vi "Add Item to Tree.vi"(8 "error in (no error)":errorcluster, 10 "Missing VI Type in":refnum<class "Missing VI Type.lvclass">, 11 "Tree Ref in":refnum<vi>) -> (0 "error out":errorcluster, 1 "Added Tag":string, 2 "Missing VI Type out":refnum<class "Missing VI Type.lvclass">, 3 "Tree Ref out":refnum<vi>)   [LabVIEW 2020, in "Peek Window.lvlib" / "Missing VI Type.lvclass"]
uses:
  Missing VI Type.lvclass
  D:/Code/VI-Peek/source/Peek Window/VI Types/Standard VI Type/Standard VI Type.lvclass
  Symbols Enum.ctl
  Standard VI Type/Standard VI Type.lvclass/Standard VI Type.ctl
  Standard VI Type/Read Full Qualified Name.vi
  Peek Window.lvlib
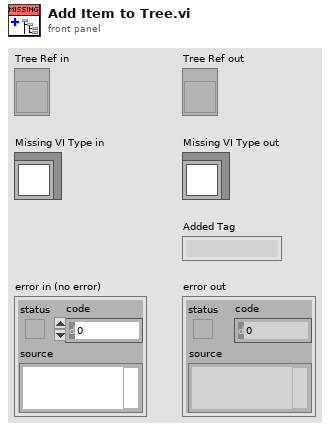
[diagram p1: front panel]
types:
  T1 = typedef "Peek Window.lvlib/Symbols Enum.ctl" = enum16{"<Blank>", "Below Here Glyph", "VI", "Dynamic Dispatch VI", "Malleable VI", "Polymorphic VI", "Missing VI", "Express VI"}
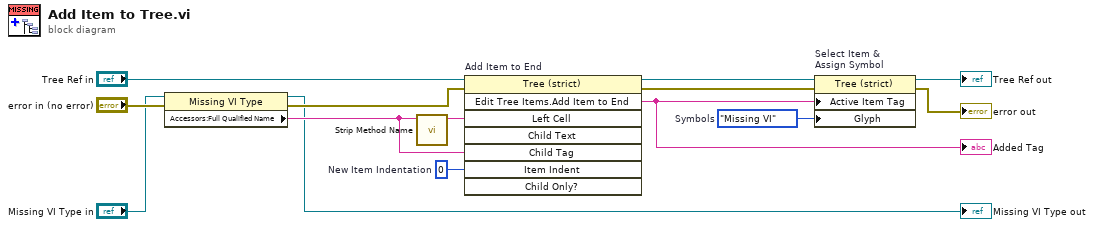
[diagram p0: block diagram]
diagram:
  w12 = Symbols_Enum."Missing VI"  # Symbols
  w14 = 0  # New Item Indentation
  n1 = property class="Missing VI Type"(reference="Missing VI Type in", error in="error in (no error)") -> (reference out=→"Missing VI Type out":refnum<class "Missing VI Type.lvclass">, error out=w7:errorcluster, "Accessors:Full Qualified Name"=w6:string)
  n2 = call "Strip Method Name.vi"("Full Qualified Name in"=w6) -> ("Plain Method Name out"=w13:string)  [unwired: 10 in]
  n3 = invoke on="Add Item to End" class="Tree (strict)" method="Edit Tree Items.Add Item to End"(reference="Tree Ref in", error in=w7, "Left Cell"=w13, "Child Tag"=w6, "Item Indent"=w14) -> (reference out=w11:refnum<vi>, error out=w8:errorcluster, "Edit Tree Items:Add Item to End"=w5:string)  [unwired: 3 in, 5 out]
  "Added Tag" <- w5
  n4 = property on="Select Item &\nAssign Symbol" class="Tree (strict)"(reference=w11, error in=w8, "Active Item Tag"=w5, "Glyph"=w12) -> (reference out=→"Tree Ref out":refnum<vi>, error out=→"error out":errorcluster)
